vi "Update Table.vi"(8 "error in (no error)":errorcluster, 10 "New Values Table":refnum<class "Basic Table.lvclass">, 11 "Basic Table in":refnum<class "Basic Table.lvclass">) -> (0 "error out":errorcluster, 3 "Basic Table out":refnum<class "Basic Table.lvclass">)   [LabVIEW 2020, in "Table.lvlib" / "Basic Table.lvclass"]
uses:
  Basic Table.lvclass
  Basic Table.lvclass/Basic Table.ctl
  <vilib>/Utility/miscctls.llb/LVMapReplaceAction.ctl
  Table Configuration Interface/Table Configuration Interface.lvclass
  Column Libraries/Column Interface/Column Interface Class/Column Interface.lvclass
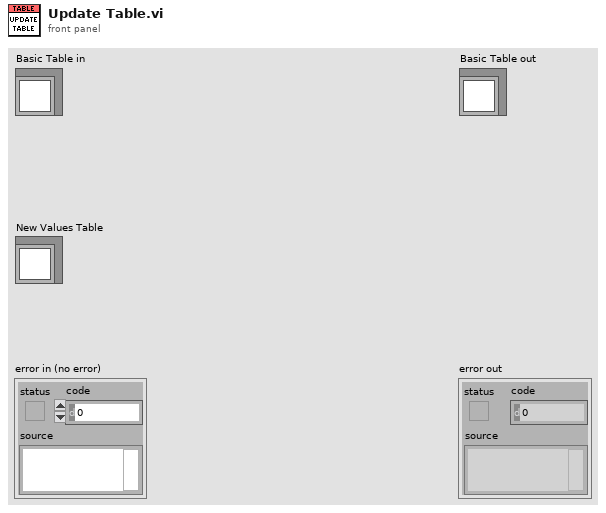
[diagram p1: front panel]
types:
  T1 = typedef "LVMapReplaceAction.ctl" = enum32{"Modify Entry only if found", "Add or Modify Entry", "Delete Entry"}
  T2 = map{string, refnum<class "Column Interface.lvclass">}
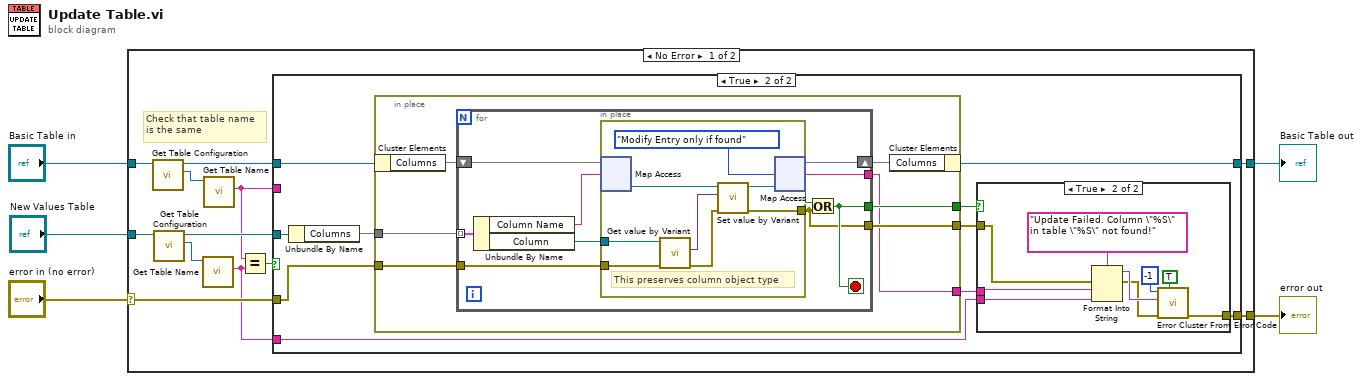
[diagram p0: block diagram]
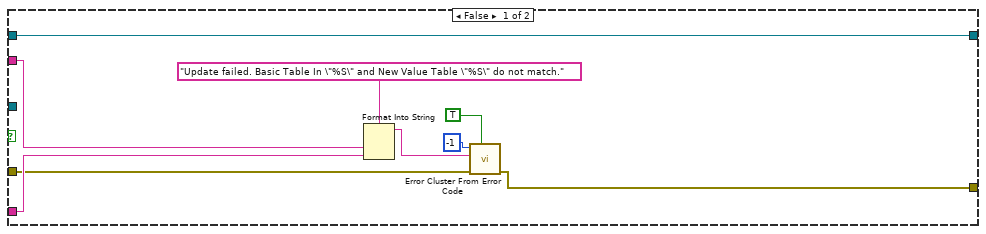
[diagram p2: hidden frame]
diagram:
  n1 = case shown="No Error" "error in (no error)" {
    selector: "error in (no error)" -> [w8 w73]
    tunnel: [w16 w73] -> w4
    tunnel: [w17 w72] -> w2
    tunnel: "Basic Table in" -> [w14 w72]
    tunnel: "New Values Table" -> [w15 _]
    frame No Error {
      # "Check that table name\nis the same"
      n2 = call "Get Table Configuration.vi"("Basic Table in"=w14) -> ("Table Configuration"=w11:refnum<class "Table Configuration Interface.lvclass">, "Basic Table out"=w13:refnum<class "Basic Table.lvclass">)  [unwired: 8 in, 1 out]
      n3 = call "Get Table Configuration.vi"("Basic Table in"=w15) -> ("Table Configuration"=w10:refnum<class "Table Configuration Interface.lvclass">, "Basic Table out"=w12:refnum<class "Basic Table.lvclass">)  [unwired: 8 in, 1 out]
      n4 = call-dynamic "Get Table Name.vi"("Table Configuration Interface in"=w10) -> ("Table Name"=w7:string)  [unwired: 8 in, 2 out]
      n5 = call-dynamic "Get Table Name.vi"("Table Configuration Interface in"=w11) -> ("Table Name"=w6:string)  [unwired: 8 in, 2 out]
      n6 = Equal?(x=w6, y=w7) -> (x = y?=w9:bool)
      n7 = case shown="True" w9 {
        tunnel: [w26 w35] -> w17
        tunnel: [w18 w32] -> w16
        tunnel: w13 -> [w26 w31]
        tunnel: w12 -> [_ w30]
        tunnel: w8 -> [w19 w29]
        tunnel: w7 -> [w23 w27]
        tunnel: w6 -> [w24 _]
        frame False {
          n8 = Format Into String(format string="Update failed. Basic Table In \"%S\" and New Value Table \"%S\" do not match.", w24, w23) -> (resulting string=w22:string)  [unwired: 2 in, 1 out]
          n9 = call <vilib>:"Error Cluster From Error Code.vi"("show call chain? (False)"=TRUE, "error in (no error)"=w19, "error message (\"\")"=w22, "error code (0)"=-1) -> ("error out"=w18:errorcluster)  [unwired: 5 in]
        }
        frame True {
          n10 = Unbundle By Name(w30) -> ("Columns"=w36:T2)
          n11 = in-place {
            in-place-border: w36 -> [w51]
            in-place-border: w29 -> [w50]
            in-place-border: [w49] -> w34
            in-place-border: [w48] -> w33
            in-place-border: [w47] -> w28
            n12 = in-place-cluster #1(w31) -> ("Columns"=w53:T2)
            n13 = for {
              tunnel: w51 -> [w62] mode=indexing
              shift-right: [w60] -> w52
              shift-left: w53 -> [w63]
              tunnel: w50 -> [w59]
              tunnel: [w57] -> w49
              tunnel: [w56] -> w48
              tunnel: [w54] -> w47
              stop <- w57 stop-if-true
              n14 = Unbundle By Name(w62) -> ("Column Name"=w55:string, "Column"=w61:refnum<class "Column Interface.lvclass">)
              n15 = in-place {
                in-place-border: w61 -> [w68]
                in-place-border: w59 -> [w66]
                in-place-border: [w64] -> w56
                # "This preserves column object type"
                n16 = in-place-map #2(w63, w55) -> (w71:refnum<class "Column Interface.lvclass">)  [unwired: 1 in, 1 out]
                n17 = call-dynamic "Get value by Variant.vi"("error in (no error)"=w66, "Column Interface in"=w68) -> ("error out"=w65:errorcluster, "Variant"=w69:variant)  [unwired: 6 in, 2 out]
                n18 = call-dynamic "Set value by Variant.vi"("error in (no error)"=w65, "Variant"=w69, "Column Interface in"=w71) -> ("error out"=w64:errorcluster, "Column Interface out"=w70:refnum<class "Column Interface.lvclass">)  [unwired: 7 in]
                n19 = in-place-map #2(w70, LVMapReplaceAction."Modify Entry only if found" ("action")) -> (w60:T2, w54:string, w58:bool)
              }
              n20 = Or(x=w58, y=w56) -> (x .or. y?=w57:bool)
            }
            n21 = in-place-cluster #1("Columns"=w52) -> (w35:refnum<class "Basic Table.lvclass">)
          }
          n22 = case shown="True" w34 {
            tunnel: w33 -> [w37 w41]
            tunnel: [w37 w42] -> w32
            tunnel: w28 -> [_ w39]
            tunnel: w27 -> [_ w38]
            frame False {
            }
            frame True {
              n23 = Format Into String(format string="Update Failed. Column \"%S\" in table \"%S\" not found!", error in=w41, w39, w38) -> (resulting string=w45:string, error out=w40:errorcluster)  [unwired: 1 in]
              n24 = call <vilib>:"Error Cluster From Error Code.vi"("show call chain? (False)"=TRUE, "error in (no error)"=w40, "error message (\"\")"=w45, "error code (0)"=-1) -> ("error out"=w42:errorcluster)  [unwired: 5 in]
            }
          }
        }
      }
    }
    frame Error {
    }
  }
  "error out" <- w4
  "Basic Table out" <- w2
